vi "PQescapeByteaConn.vi"(6 "error in (no error)":errorcluster, 8 "to_length":u32, 9 "from_length":u32, 10 "from":string, 11 "conn":u32) -> (0 "to_length out":u32, 1 "from_out":string, 2 "PQescapeByteaConn":string, 3 "conn_out":u32, 4 "error out":errorcluster)   [LabVIEW 2019, in "libpqlv.lvlib"]
uses:
  libpqlv.lvlib
  libpq.dll
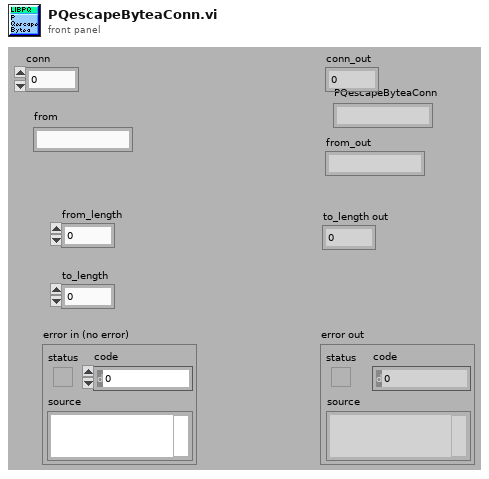
[diagram p1: front panel]
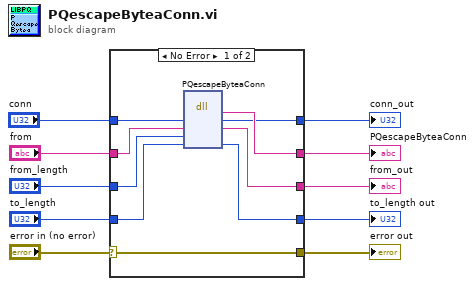
[diagram p0: block diagram]
diagram:
  n1 = case shown="No Error" "error in (no error)" {
    selector: "error in (no error)" -> [w19 w23]
    tunnel: [w19 w23] -> w9
    tunnel: [w18 _] -> w8
    tunnel: [w17 w21] -> w3
    tunnel: "from" -> [w16 w20]
    tunnel: "from_length" -> [w15 _]
    tunnel: "to_length" -> [w14 w22]
    tunnel: [w13 w22] -> w4
    tunnel: "conn" -> [w12 w21]
    tunnel: [w11 w20] -> w1
    frame No Error {
      n2 = dll-call lib="libpq.*" fn="PQescapeByteaConn"("conn"=w12, "from"=w16, "from_length"=w15, "to_length"=w14) -> ("PQescapeByteaConn"=w18:string, "conn"=w17:u32, "from"=w11:string, "to_length"=w13:u32)  [unwired: 4 in, 2 out]
    }
    frame Error {
    }
  }
  "PQescapeByteaConn" <- w8
  "to_length out" <- w4
  "error out" <- w9
  "conn_out" <- w3
  "from_out" <- w1
